vi "Evaluate Loaded Stats.vi"(6 "CMDCluster In":T1, 8 "Data Array":string[][](array[string]), 11 "Stat Array In":string[][](array[string])) -> (0 "Invalid?":bool, 3 "Stat Array Out":string[][](array[string]))   [LabVIEW 2013]
uses:
  TypeDef/Command Cluster.ctl
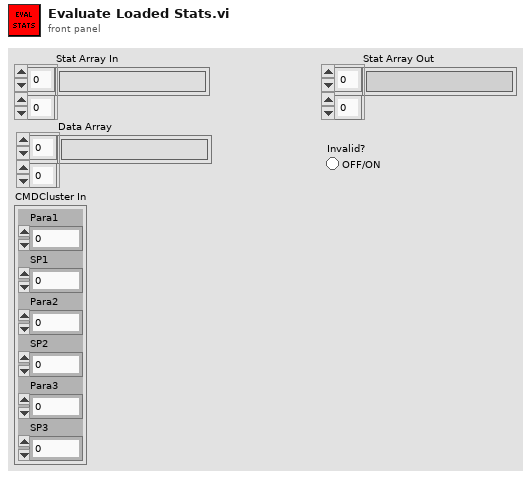
[diagram p1: front panel]
types:
  T1 = typedef "Command Cluster.ctl" = cluster{"Para1":i32, "SP1":dbl, "Para2":i32, "SP2":dbl, "Para3":i32, "SP3":dbl}
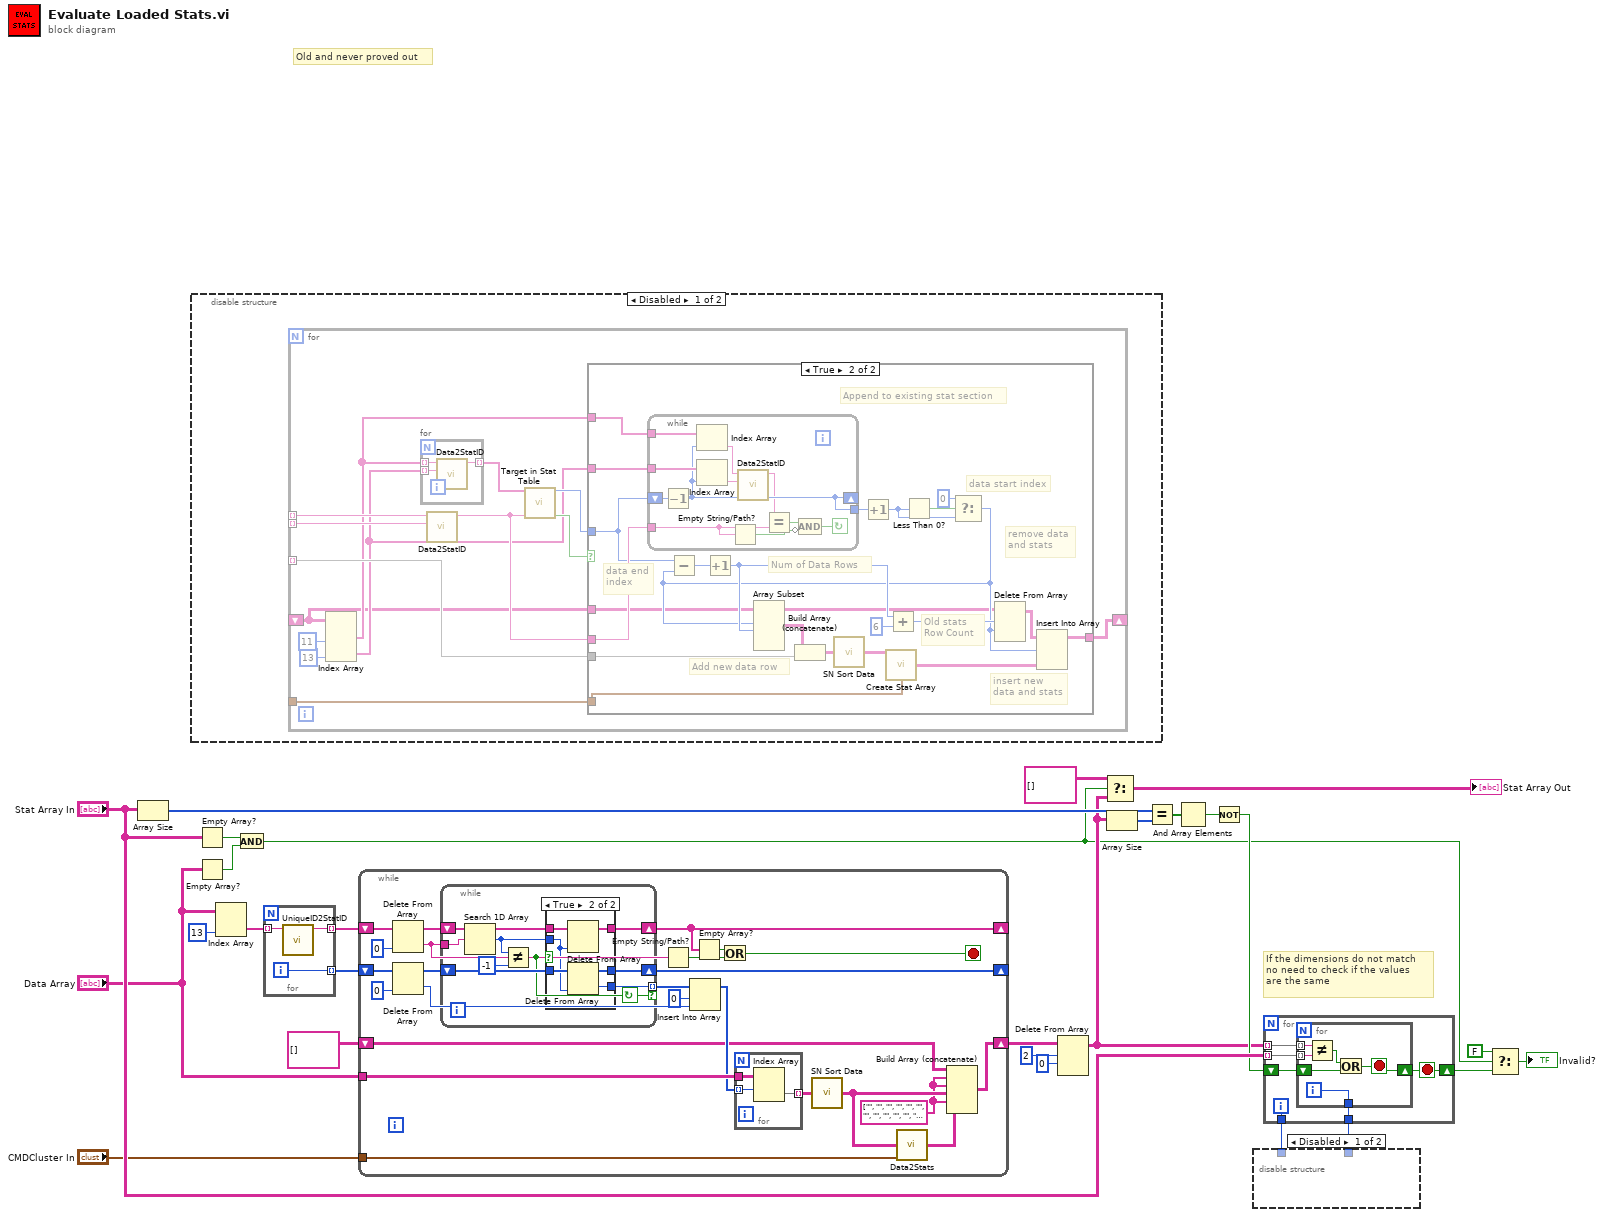
[diagram p0: block diagram]
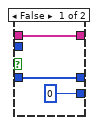
[diagram p3: hidden frame]
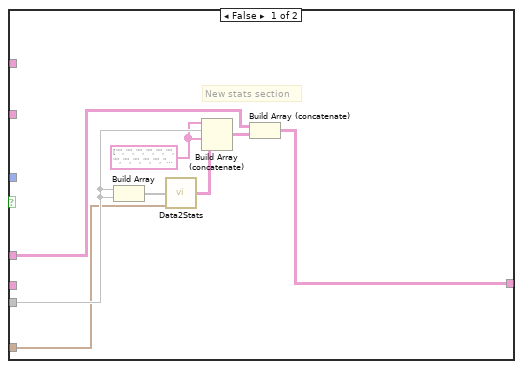
[diagram p4: hidden frame]
diagram:
  # "Old and never proved out"
  # "If the dimensions do not match\nno need to check if the values\nare the same"
  n1 = Array Size(array="Stat Array In") -> (size(s)=w24:i32[])
  n2 = disable-structure shown="Disabled" {
    frame Disabled {
      n3 = for {
        tunnel: _ -> [w39] mode=indexing
        tunnel: _ -> [w36] mode=indexing
        shift-right: [w38] -> _
        shift-left: _ -> [w28]
        tunnel: _ -> [w37]
        tunnel: _ -> [w35] mode=indexing
        n4 = Index Array(array=w28, index (col) #1=11 ("disabled index (col)"), index (col) #2=13 ("index (col)")) -> (element #1=w30:string[], element #2=w29:string[])  [unwired: 2 in]
        n5 = for {
          tunnel: w30 -> [w44] mode=indexing
          tunnel: w29 -> [w43] mode=indexing
          tunnel: [w42] -> w31 mode=indexing
          n6 = call "Data2StatID.vi"("ParameterSet"=w43, "Step"=w44) -> ("StatID"=w42:string)  [unwired: 9 in]
        }
        n7 = call "Data2StatID.vi"("ParameterSet"=w36, "Step"=w35) -> ("StatID"=w34:string)  [unwired: 9 in]
        n8 = call "Target in Stat Table.vi"("Stat ID Column"=w31, "Target Parameters"=w34) -> ("LastDataIndex"=w41:i32, "TargetInStats"=w40:bool)  [unwired: 12 in]
        n9 = case shown="True" w40 {
          tunnel: w41 -> [_ w68]
          tunnel: w39 -> [w52 w72]
          tunnel: [w51 w69] -> w38
          tunnel: w34 -> [_ w73]
          tunnel: w29 -> [_ w74]
          tunnel: w37 -> [w46 w55]
          tunnel: w30 -> [_ w54]
          tunnel: w28 -> [w45 w53]
          frame False {
            w49 = string[] ["", "", "", "", "", "", "", "", "", "", "", "", "", ""]
            # "New stats section"
            n10 = Build Array(w52, w52) -> (w48:void[])
            n11 = call "Data2Stats.vi"("DataIn"=w48, "CMDCluster In"=w46) -> ("StatsOut"=w47:string[][])  [unwired: 13 in]
            n12 = Build Array (concatenate)(w49, w52, w49, w47) -> (w50:string[][])
            n13 = Build Array (concatenate)(w45, w50) -> (w51:string[][])
          }
          frame True {
            # "Append to existing stat section"
            # "insert new\ndata and stats"
            # "remove data\nand stats"
            # "Add new data row"
            # "Old stats\nRow Count"
            # "Num of Data Rows"
            # "data start index"
            # "data end\nindex"
            n14 = while {
              tunnel: w74 -> [w84]
              tunnel: w73 -> [w76]
              shift-right: [w82] -> _
              shift-left: w68 -> [w85]
              tunnel: [w82] -> w62
              tunnel: w54 -> [w83]
              stop <- w75 continue-if-true
              n15 = Decrement(x=w85) -> (x-1=w82:i32)
              n16 = Index Array(array=w83, index=w82) -> (element=w80:string)
              n17 = Index Array(array=w84, index=w82) -> (element=w81:string)
              n18 = Empty String/Path?(string/path=w76) -> (empty?=w77:bool)
              n19 = call "Data2StatID.vi"("ParameterSet"=w81, "Step"=w80) -> ("StatID"=w79:string)  [unwired: 9 in]
              n20 = Equal?(x=w79, y=w76) -> (x = y?=w78:bool)
              n21 = Compound Arithmetic op=AND(w78, invert w77) -> (w75:bool)
            }
            n22 = Increment(x=w62) -> (x+1=w61:i32)
            n23 = Less Than 0?(x=w61) -> (x < 0?=w66:bool)
            n24 = Select(t=0, s=w66, f=w61) -> (s? t:f=w58:i32)
            n25 = Subtract(x=w68, y=w58) -> (x-y=w64:i32)
            n26 = Increment(x=w64) -> (x+1=w63:i32)
            n27 = Array Subset(array=w53, index (row)=w58, length (row)=w63) -> (w67:string[][])  [unwired: 2 in]
            n28 = Build Array (concatenate)(w67, w72) -> (w57:string[][])
            n29 = call "SN Sort Data.vi"("Array In"=w57) -> ("Array Out"=w56:string[][])  [unwired: 13 in, 1 out]
            n30 = call "Create Stat Array.vi"("DataIn"=w56, "CommandCluster"=w55) -> ("StatArray"=w60:string[][])  [unwired: 13 in]
            n31 = Add(x=w63, y=6) -> (x+y=w59:i32)
            n32 = Delete From Array(array=w53, length=w59, index (row)=w58) -> (array with subset deleted=w70:string[][])  [unwired: 1 in, 1 out]
            n33 = Insert Into Array(array=w70, index (row)=w58, new element=w60) -> (w69:string[][])  [unwired: 1 in]
          }
        }
      }
    }
    frame Enabled {
    }
  }
  n34 = Empty Array?(array="Stat Array In") -> (empty?=w25:bool)
  n35 = Empty Array?(array="Data Array") -> (empty?=w18:bool)
  n36 = Index Array(array="Data Array", index (col)=13 ("disabled index (col)")) -> (element=w4:string[])  [unwired: 1 in]
  n37 = And(x=w25, y=w18) -> (x .and. y?=w9:bool)
  n38 = for {
    tunnel: w4 -> [w86] mode=indexing
    tunnel: [w88] -> w16 mode=indexing
    tunnel: [w87] -> w5 mode=indexing
    i -> [w88]
    n39 = call "UniqueID2StatID.vi"("UniqueID"=w86) -> ("StatID"=w87:string)  [unwired: 10 in]
  }
  n40 = while {
    shift-right: [w95] -> _
    shift-left: w5 -> [w112]
    shift-right: [w103] -> _
    shift-left: w16 -> [w108]
    shift-right: [w91] -> w11
    shift-left: string[][] [] -> [w90]
    tunnel: "CMDCluster In" -> [w101]
    tunnel: "Data Array" -> [w99]
    stop <- w92 stop-if-true
    w89 = string[] ["", "", "", "", "", "", "", "", "", "", "", "", "", ""]
    n41 = Delete From Array(array=w112, index=0) -> (deleted portion=w96:string, array with subset deleted=w110:string[])  [unwired: 1 in]
    n42 = Delete From Array(array=w108, index=0) -> (deleted portion=w105:i32, array with subset deleted=w107:i32[])  [unwired: 1 in]
    n43 = while {
      shift-right: [w119] -> w95
      shift-left: w110 -> [w122]
      shift-right: [w118] -> w103
      shift-left: w107 -> [w120]
      tunnel: w96 -> [w124]
      tunnel: [w117] -> w104 mode=indexing if=w116
      stop <- w116 continue-if-true
      n44 = Search 1D Array(1D array=w122, element=w124) -> (index of element=w121:i32)  [unwired: 1 in]
      n45 = Not Equal?(x=w121, y=-1) -> (x != y?=w116:bool)
      n46 = case shown="True" w116 {
        tunnel: w122 -> [w127 w133]
        tunnel: w121 -> [_ w128]
        tunnel: w120 -> [w126 w132]
        tunnel: [w127 w131] -> w119
        tunnel: [w126 w130] -> w118
        tunnel: [0 w129] -> w117
        frame False {
        }
        frame True {
          n47 = Delete From Array(array=w133, index=w128) -> (array with subset deleted=w131:string[])  [unwired: 1 in, 1 out]
          n48 = Delete From Array(array=w132, index=w128) -> (deleted portion=w129:i32, array with subset deleted=w130:i32[])  [unwired: 1 in]
        }
      }
    }
    n49 = Empty String/Path?(string/path=w96) -> (empty?=w93:bool)
    n50 = Insert Into Array(array=w104, index=0, new element=w105) -> (w98:i32[])
    n51 = Empty Array?(array=w95) -> (empty?=w94:bool)
    n52 = Or(x=w94, y=w93) -> (x .or. y?=w92:bool)
    n53 = for {
      tunnel: w99 -> [w115]
      tunnel: w98 -> [w114] mode=indexing
      tunnel: [w113] -> w97 mode=indexing
      n54 = Index Array(array=w115, index (row)=w114) -> (element=w113:string[])  [unwired: 1 in]
    }
    n55 = call "SN Sort Data.vi"("Array In"=w97) -> ("Array Out"=w100:string[][])  [unwired: 13 in, 1 out]
    n56 = call "Data2Stats.vi"("DataIn"=w100, "CMDCluster In"=w101) -> ("StatsOut"=w102:string[][])  [unwired: 13 in]
    n57 = Build Array (concatenate)(w90, w89, w89, w100, w89, w102) -> (w91:string[][])
  }
  n58 = Delete From Array(array=w11, length=2, index (row)=0) -> (array with subset deleted=w10:string[][])  [unwired: 1 in, 1 out]
  n59 = Select(t=string[][] [], s=w9, f=w10) -> (s? t:f=→"Stat Array Out":string[][])
  n60 = Array Size(array=w10) -> (size(s)=w23:i32[])
  n61 = Equal?(x=w24, y=w23) -> (x = y?=w22:bool[])
  n62 = And Array Elements(Boolean array=w22) -> (logical AND=w20:bool)
  n63 = Not(x=w20) -> (.not. x?=w19:bool)
  n64 = for {
    tunnel: w10 -> [w139] mode=indexing
    tunnel: "Stat Array In" -> [w138] mode=indexing
    shift-right: [w136] -> w8
    shift-left: w19 -> [w137]
    tunnel: [w135] -> w2
    tunnel: [w134] -> w1
    i -> [w135]
    stop <- w136 stop-if-true
    n65 = for {
      tunnel: w139 -> [w145] mode=indexing
      tunnel: w138 -> [w144] mode=indexing
      shift-right: [w141] -> w136
      shift-left: w137 -> [w143]
      tunnel: [w140] -> w134
      i -> [w140]
      stop <- w141 stop-if-true
      n66 = Not Equal?(x=w145, y=w144) -> (x != y?=w142:bool)
      n67 = Or(x=w142, y=w143) -> (x .or. y?=w141:bool)
    }
  }
  n68 = disable-structure shown="Disabled" {
    disable-tunnel: w2 -> [_ _]
    disable-tunnel: w1 -> [_ _]
    frame Disabled {
    }
    frame Enabled {
    }
  }
  n69 = Select(t=FALSE, s=w9, f=w8) -> (s? t:f=→"Invalid?":bool)
